vi "Daten weitergeben.vi"(6 "Aktionen":T1, 8 "Antwort":string, 9 "Empfangspuffer":string, 11 "Detail":string) -> (0 "Antwort":string[](array[string]), 1 "Empfangspuffer":string[](array[string]), 2 "Details ALLE":string[](array[string]), 3 "Log Daten":string[](array[string]), 5 "Details":string[](array[string]))   [LabVIEW 2020, in "AK-Schnittstelle.lvlib"]
uses:
  AK-Schnittstelle.lvlib
  Daten weitergeben Aktionen.ctl
  Allgemein/allgemeine Sub-VIs.lvlib
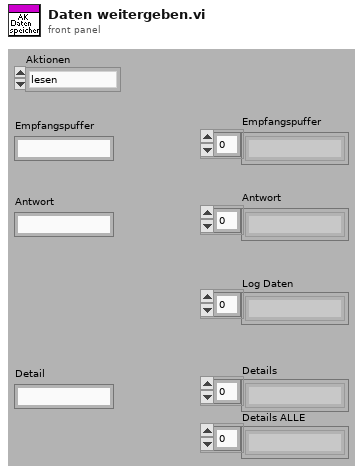
[diagram p1: front panel]
types:
  T1 = typedef "AK-Schnittstelle.lvlib/Daten weitergeben Aktionen.ctl" = enum16{"lesen", "schreiben", "Log löschen", "Detail", "Detail löschen", "Speicher Freigeben"}
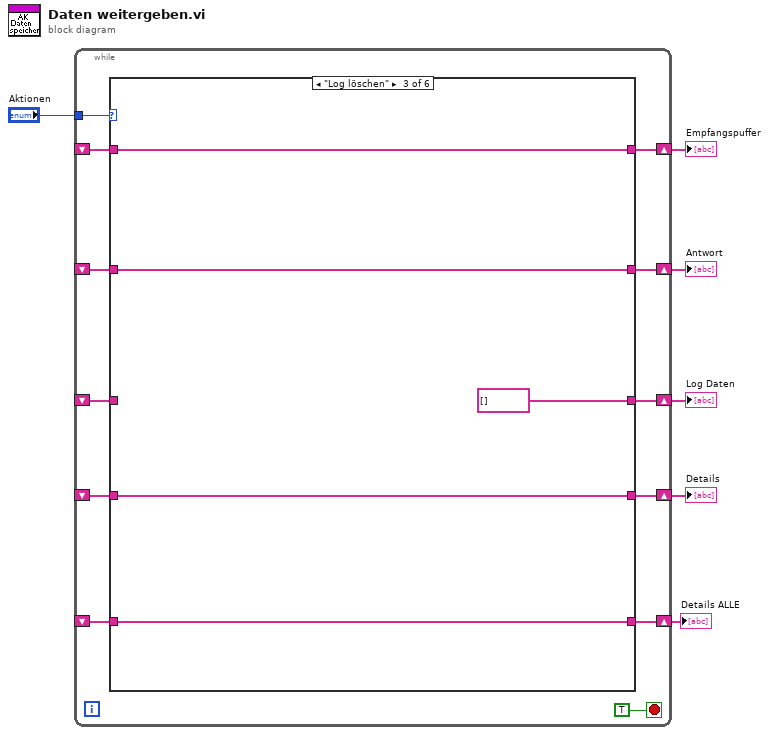
[diagram p0: block diagram]
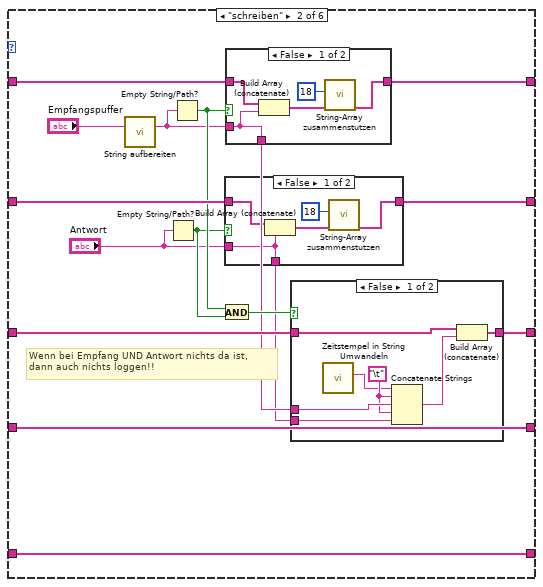
[diagram p3: hidden frame]
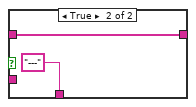
[diagram p5: hidden frame]
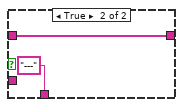
[diagram p6: hidden frame]
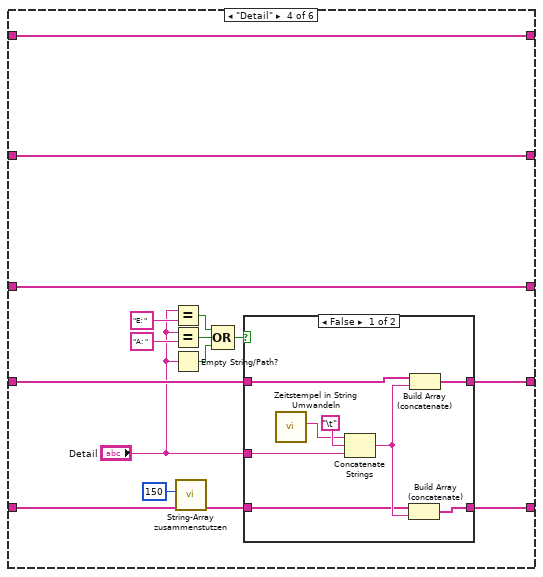
[diagram p7: hidden frame]
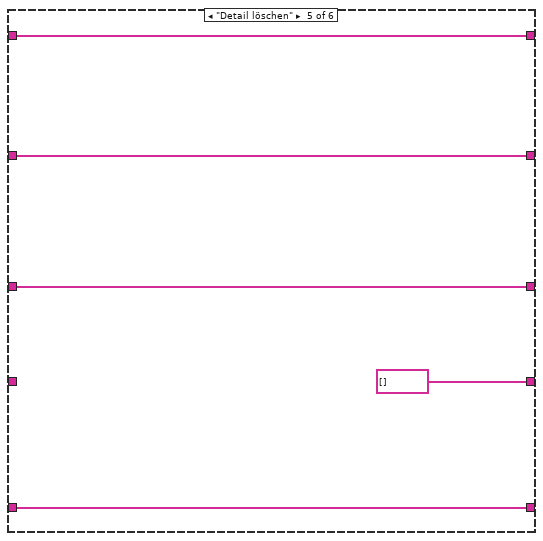
[diagram p9: hidden frame]
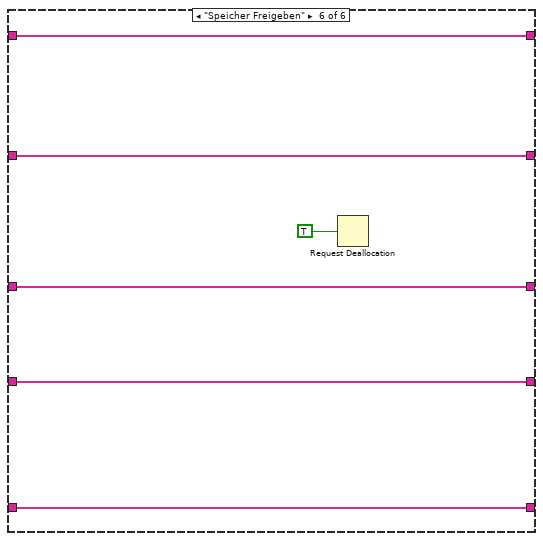
[diagram p10: hidden frame]
diagram:
  n1 = while {
    shift-right: [w16] -> w5
    shift-left: _ -> [w14]
    shift-right: [w15] -> w4
    shift-left: _ -> [w13]
    tunnel: "Aktionen" -> [w17]
    shift-right: [w12] -> w3
    shift-left: _ -> [w11]
    shift-right: [w10] -> w2
    shift-left: _ -> [w9]
    shift-right: [w8] -> w1
    shift-left: _ -> [w7]
    stop <- TRUE stop-if-true
    n2 = case shown="\"Log löschen\"" w17 {
      tunnel: [w23 w39 w66 w82 w97 w103] -> w16
      tunnel: [w22 w37 w65 w81 w96 w102] -> w15
      tunnel: w14 -> [w23 w38 w66 w82 w97 w103]
      tunnel: w13 -> [w22 w36 w65 w81 w96 w102]
      tunnel: [w21 w29 string[] [] w80 w94 w101] -> w12
      tunnel: w11 -> [w21 w28 _ w80 w94 w101]
      tunnel: [w20 w25 w63 w71 string[] [] w100] -> w10
      tunnel: w9 -> [w20 w25 w63 w79 _ w100]
      tunnel: [w19 w24 w62 w70 w93 w99] -> w8
      tunnel: w7 -> [w19 w24 w62 w68 w93 w99]
      frame "lesen", Default {
      }
      frame "schreiben" {
        # "Wenn bei Empfang UND Antwort nichts da ist, \ndann auch nichts loggen!!"
        n3 = call "String aufbereiten.vi"("read buffer"="Empfangspuffer") -> ("String"=w31:string)  [unwired: 14 in]
        n4 = Empty String/Path?(string/path="Antwort") -> (empty?=w33:bool)
        n5 = Empty String/Path?(string/path=w31) -> (empty?=w34:bool)
        n6 = And(x=w34, y=w33) -> (x .and. y?=w32:bool)
        n7 = case shown="False" w33 {
          tunnel: w36 -> [w52 w54]
          tunnel: [w49 w54] -> w37
          tunnel: "Antwort" -> [w48 _]
          tunnel: [w48 "---" ("String")] -> w26
          frame False {
            n8 = Build Array (concatenate)(w52, w48) -> (w51:string[])
            n9 = call "String-Array zusammenstutzen.vi"("Array"=w51, "Anzahl Elemente"=18) -> ("Array"=w49:string[])  [unwired: 9 in]
          }
          frame True {
          }
        }
        n10 = case shown="False" w34 {
          tunnel: w38 -> [w59 w61]
          tunnel: [w56 w61] -> w39
          tunnel: w31 -> [w55 _]
          tunnel: [w55 "---" ("String")] -> w27
          frame False {
            n11 = Build Array (concatenate)(w59, w55) -> (w58:string[])
            n12 = call "String-Array zusammenstutzen.vi"("Array"=w58, "Anzahl Elemente"=18) -> ("Array"=w56:string[])  [unwired: 9 in]
          }
          frame True {
          }
        }
        n13 = case shown="False" w32 {
          tunnel: w27 -> [w46 _]
          tunnel: w26 -> [w45 _]
          tunnel: [w43 w47] -> w29
          tunnel: w28 -> [w40 w47]
          frame False {
            w42 = "\t"
            n14 = call "Zeitstempel in String Umwandeln.vi"() -> ("Zeitstempel mit Kommastellen"=w41:string)  [unwired: 10 in, 1 out]
            n15 = Concatenate Strings(w41, w42, w46, w42, w45) -> (w44:string)
            n16 = Build Array (concatenate)(w40, w44) -> (w43:string[])
          }
          frame True {
          }
        }
      }
      frame "Log löschen" {
      }
      frame "Detail" {
        n17 = Equal?(x="Detail", y="E: " ("String")) -> (x = y?=w72:bool)
        n18 = Equal?(x="Detail", y="A: " ("String")) -> (x = y?=w75:bool)
        n19 = Empty String/Path?(string/path="Detail") -> (empty?=w74:bool)
        n20 = call "String-Array zusammenstutzen.vi"("Array"=w68, "Anzahl Elemente"=150) -> ("Array"=w67:string[])  [unwired: 9 in]
        n21 = Compound Arithmetic op=OR(w72, w75, w74) -> (w73:bool)
        n22 = case shown="False" w73 {
          tunnel: "Detail" -> [w90 _]
          tunnel: [w89 w92] -> w71
          tunnel: w79 -> [w86 w92]
          tunnel: [w84 w91] -> w70
          tunnel: w67 -> [w83 w91]
          frame False {
            n23 = call "Zeitstempel in String Umwandeln.vi"() -> ("Zeitstempel mit Kommastellen"=w87:string)  [unwired: 10 in, 1 out]
            n24 = Concatenate Strings(w87, "\t", w90) -> (w85:string)
            n25 = Build Array (concatenate)(w83, w85) -> (w84:string[])
            n26 = Build Array (concatenate)(w86, w85) -> (w89:string[])
          }
          frame True {
          }
        }
      }
      frame "Detail löschen" {
      }
      frame "Speicher Freigeben" {
        n27 = Request Deallocation(TRUE ("Flag")) -> ()
      }
    }
  }
  "Empfangspuffer" <- w5
  "Antwort" <- w4
  "Log Daten" <- w3
  "Details" <- w2
  "Details ALLE" <- w1
